vi "findInCompiledList.vi"(8 "error in (no error)":errorcluster, 9 "Path":path, 11 "ExperimentRunner in":refnum<class "ExperimentRunner.lvclass">) -> (0 "error out":errorcluster, 3 "ExperimentRunner out":refnum<class "ExperimentRunner.lvclass">)   [LabVIEW 2009, in "Views.lvlib" / "ExperimentControl.lvlib" / "ExperimentRunner.lvclass"]
uses:
  ExperimentRunner.lvclass
  ExperimentRunner.lvclass/ExperimentRunner.ctl
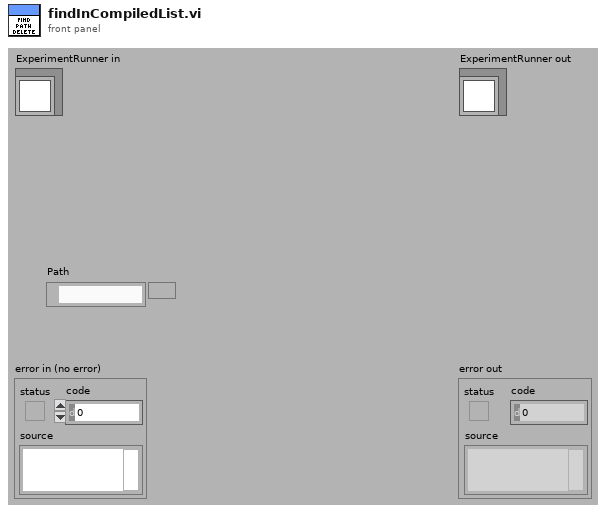
[diagram p1: front panel]
types:
  T1 = cluster{"CompilerPath":path, "CompilerString":string}[]
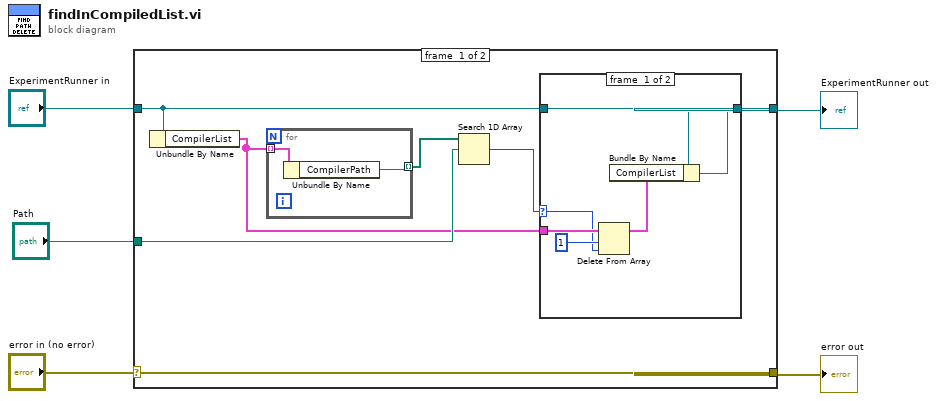
[diagram p0: block diagram]
diagram:
  n1 = case shown="No Error" "error in (no error)" {
    selector: "error in (no error)" -> [w12 w23]
    tunnel: [w12 w23] -> w4
    tunnel: [w7 w22] -> w2
    tunnel: "ExperimentRunner in" -> [w8 w22]
    tunnel: "Path" -> [w10 _]
    frame #0 {
      n2 = Unbundle By Name(w8) -> ("CompilerList"=w6:T1)
      n3 = for {
        tunnel: w6 -> [w21] mode=indexing
        tunnel: [w20] -> w11 mode=indexing
        n4 = Unbundle By Name(w21) -> ("CompilerPath"=w20:path)
      }
      n5 = Search 1D Array(1D array=w11, element=w10) -> (index of element=w9:i32)  [unwired: 1 in]
      n6 = case shown="0, Default" w9 {
        selector: w9 -> [w16 _]
        tunnel: w8 -> [w15 w19]
        tunnel: [w14 w19] -> w7
        tunnel: w6 -> [w18 _]
        frame #0 {
          n7 = Delete From Array(array=w18, length=1, index=w16) -> (array with subset deleted=w13:T1)  [unwired: 1 out]
          n8 = Bundle By Name(cluster=w15, "CompilerList"=w13) -> (w14:refnum<class "ExperimentRunner.lvclass">)
        }
        frame #1 {
          # "not found"
        }
      }
    }
    frame #1 {
    }
  }
  "error out" <- w4
  "ExperimentRunner out" <- w2
